vi "ZS_DPLab_Main_ver4.0.vi"() -> ()   [LabVIEW 2012]
panel:
  in  "File type":u16(ring) items=["Txt"=0, "Both"=2]
  out "StartTime(ms)":u32
  in  "Pause":bool
  in  "stop":bool
  in  "Main Sweep":u8(ring) items=["Time", "DC Current", "Delta Current", "Pulse Delta Current", "Sine Current", "Lock-In Vosc"]
  out "Run index":string
  in  "File Index:":u16=1 format="%03d"
  out "TakingData":bool
  in  "Data File Address":path
  in  "Tab Control":T1(tab)
  in  "Steps Config:":T2={"# of points:"=100, "Step Delay (s)"=1.0, "Ini Delay (s)"=3.0, "# of steps:"=1} {"# of steps:" step=1; "# of points:" step=1; "Step Delay (s)" min=0.0 format="%3.2f"; "Ini Delay (s)" min=0.0 format="%3.2f"}
  in  "Tab Control 2":enum32{"ITC 503", "LS 340"}(tab)
  in  "Temperature Control (ITC 503):":T3={"GPIB ADR"=0, "Change Heater?"={"Change Heater?"=FALSE, "Heater"=0}, "Change Temp?"={"Change Temp?"=FALSE, "Set Temp (K)"=0.0}, "Cluster"={"Heat Auto?"=FALSE, "Manual Heat?"=FALSE, "Heater Manual (%)"=0.0}, "Change PID?"={"Change PID?"=FALSE, "Proportional"=0.0, "Integral"=0.0, "Derivative"=0.0}, "Change Para?"=FALSE, "ITC503 Control Sensor"=1} {"ITC503 Control Sensor" items=["T2", "T3"]; "Change PID?"."Derivative" format="%.2f"; "Change PID?"."Integral" format="%.2f"; "Change PID?"."Proportional" format="%.2f"; "Cluster"."Heater Manual (%)" scale=0.0..100.0; "Change Temp?"."Set Temp (K)" format="%.3f"; "Change Heater?"."Heater" items=["Heater 1", "Heater 2", "Heater 3"]; "GPIB ADR" items=["None"=0, "24"=24]}
  in  "Temperature Control (LS 340):":T4={"GPIB ADR"=0, "From (K)"=0.0, "To (K)"=0.0, "Rate (K/min; 0~100)"=1.0, "Delta T (0.08K)"=0.08, "Temp. Header"="Temp_K", "Temp. Display controller"={"Ch B"=TRUE, "Ch C"=TRUE, "Ch D"=FALSE}} {"Delta T (0.08K)" format="%.3f"; "Rate (K/min; 0~100)" format="%.1f"; "To (K)" format="%.2f"; "From (K)" format="%.3f"; "GPIB ADR" items=["None"=0, "30"=30, "12"=12]}
  in  "Measuring Instruments :":T5(array[cluster])
  in  "Keithley 6221 :":T6(array[cluster]) {"Sweep Mode" items=["Linear", "Log", "Exp", "Inverse", "Manual"]; "GPIB ADR" items=["None"=0, "12"=12, "13"=13]; "To I_Sin (A)" format="%#.5p"; "To I_H (A)" format="%#.5p"; "To I_HI (A)" format="%#.5p"; "To I (A)" format="%#.5p"; "Delay (s)" format="%.3p"; "Pulse Width (s)" format="%.3p"; "Delay Time (s)" format="%#.5p"; "DC Offset (A)" format="%#.5p"; "From I_Sin (A)" format="%#.5p"; "Freq (Hz)" format="%#_6p"; "I_L (A)" format="%#.5p"; "From I_H (A)" format="%#.5p"; "I_LO (A)" format="%#.5p"; "From I (A)" format="%#.5p"; "From I_HI (A)" format="%#.5p"}
  in  "Lock-In SR7265 :":T7(array[cluster]) {"Sweep Mode" items=["Linear", "Log", "Exp", "Inverse", "Manual"]; "To" format="%#.5p"; "From" format="%#.5p"; "GPIB ADR" items=["None"=0, "11"=11, "16"=16]}
  in  "Description of this measurement":string
  in  "Varialbe Instruments:":i32(listbox)
  in  "Instruments Config:":string[][](table) caption="Table"
  out "Configuration Profile:":string
  in  "Up Button":bool
  in  "Delete Button":bool
  in  "Down Button":bool
  in  "Add one Run":bool
  in  "Tab Control 3":enum32{"ReadMe", "IPS120", "CS4"}(tab)
  in  "Magnet Control (IPS 120-10)":T8={"Action"=1, "Standby (s)"=0.0, "Heater on (s)"=300.0, "Sweep Setup "=[], "GPIB ADR"=0, "Change Para?"=FALSE} {"GPIB ADR" items=["None"=0, "25"=25]; "Sweep Setup"."Hold(min)" min=0.0; "Sweep Setup"."Set Rate(T/min)" min=0.001 max=0.5 step=0.001; "Sweep Setup"."Set Point (T)" min=-9.0 max=9.0 step=0.001; "Action" items=["Hold", "To Set Point", "To Zero", "Clamp"]}
  in  "Magnet Control (CS4)":T9={"Action"=1, "Standby (s)"=0.0, "Heater on (s)"=300.0, "Sweep Setup "=[], "GPIB ADR"=0, "Change Para?"=FALSE} {"GPIB ADR" items=["None"=0, "10"=10]; "Sweep Setup"."Rate in Range (T/min)" min=0.001 max=0.5 step=0.001 format="%_6g"; "Sweep Setup"."Hold(min)" min=0.0; "Sweep Setup"."Set Point (T)" min=-12.0 max=12.0 step=0.001; "Action" items=["Up", "Down", "Pause", "Zero"]}
  in  "SettingGo":bool
  in  "Discarded pts":i32
  in  "Analysis":bool=TRUE
  in  "Measure with H/T sweep?":bool=TRUE
  in  "LS372 Bridge :":T10(array[cluster]) {"Voltage" items=["2.00 uV"=1, "6.32 uV"=2, "20.0 uV"=3, "63.2 uV"=4, "200 uV"=5, "632 uV"=6, "2.0 mV"=7, "6.32 mV"=8]; "Current" items=["1.00 pA"=1, "3.16 pA"=2, "10.0 pA"=3, "31.6 pA"=4, "100 pA"=5, "316 pA"=6, "1.00 nA"=7, "3.16 nA"=8, "10 nA"=9, "31.6 nA"=10, "100 nA"=11, "316 nA"=12, "1.00 uA"=13, "3.16 uA"=14, "10.0 uA"=15, "31.6 uA"=16, "100 uA"=17, "316 uA"=18, "1.00 mA"=19, "3.16 mA"=20, "10.0 mA"=21, "31.6 mA"=22]; "Range (Ohms)" items=["2.0 m"=1, "6.32 m"=2, "20.0 m"=3, "63.2 m"=4, "200 m"=5, "632 m"=6, "2.00"=7, "6.32"=8, "20.0"=9, "63.2"=10, "200"=11, "632"=12, "2.00 k"=13, "6.32 k"=14, "20.0 k"=15, "63.2 k"=16, "200 k"=17, "632 k"=18, "2.00 M"=19, "6.32 M"=20, "20.0 M"=21, "63.2 M"=22]; "Excitation Mode" items=["Voltage", "Current"]; "GPIB ADR" items=["3"=3, "None"=0, "9"=9]}
  in  "Run Batch Array":T11(array[cluster]) {"Magnet Control (CS4) 2"."GPIB ADR" items=["None"=0, "25"=25]; "Magnet Control (CS4) 2"."Sweep Setup"."Rate in Range (T/min)" min=0.001 max=0.5 step=0.001; "Magnet Control (CS4) 2"."Sweep Setup"."Hold(min)" min=0.0; "Magnet Control (CS4) 2"."Sweep Setup"."Set Point (T)" min=-9.0 max=9.0 step=0.001; "Magnet Control (CS4) 2"."Action" items=["Up", "Down", "Pause", "Zero"]; "LS372 Bridge : 2"."Voltage" items=["2.00 uV"=1, "6.32 uV"=2, "20.0 uV"=3, "63.2 uV"=4, "200 uV"=5, "632 uV"=6, "2.0 mV"=7, "6.32 mV"=8]; "LS372 Bridge : 2"."Current" items=["1.00 pA"=1, "3.16 pA"=2, "10.0 pA"=3, "31.6 pA"=4, "100 pA"=5, "316 pA"=6, "1.00 nA"=7, "3.16 nA"=8, "10 nA"=9, "31.6 nA"=10, "100 nA"=11, "316 nA"=12, "1.00 uA"=13, "3.16 uA"=14, "10.0 uA"=15, "31.6 uA"=16, "100 uA"=17, "316 uA"=18, "1.00 mA"=19, "3.16 mA"=20, "10.0 mA"=21, "31.6 mA"=22]; "LS372 Bridge : 2"."Range" items=["2.0 m"=1, "6.32 m"=2, "20.0 m"=3, "63.2 m"=4, "200 m"=5, "632 m"=6, "2.00"=7, "6.32"=8, "20.0"=9, "63.2"=10, "200"=11, "632"=12, "2.00 k"=13, "6.32 k"=14, "20.0 k"=15, "63.2 k"=16, "200 k"=17, "632 k"=18, "2.00 M"=19, "6.32 M"=20, "20.0 M"=21, "63.2 M"=22]; "LS372 Bridge : 2"."Excitation" items=["Voltage", "Current"]; "LS372 Bridge : 2"."GPIB" items=["None"=0, "9"=9]; "Main Sweep" items=["Time", "DC Current", "Delta Current", "Pulse Delta Current", "Sine Current", "Lock-in Vosc"]; "Temperature Control (ITC 503):"."Sensor" items=["T2", "T3"]; "Magnet Control (IPS 120-10)"."Action" items=["Hold", "To Set point", "To Zero", "Clamp"]; "Keithley 6221 :"."Sweep Mode" items=["Linear", "Log", "Exp", "Inverse", "Manual"]}
  in  "Delete Run":bool
  in  "BatchSettingGo":bool
  out "T2":string
  out "T3":string
  out "B":string
  out "T1":string
  in  "DisplayControl":T12 {"Scale" items=["L", "R"]; "Y - axes"."Y 6" items=["", "Time_sec", "Temp_K", "ChC_K", "BField_T", "Rx", "Ry", "Rx", "Ry"]; "Y - axes"."Y 5" items=["", "Time_sec", "Temp_K", "ChC_K", "BField_T", "Rx", "Ry", "Rx", "Ry"]; "Y - axes"."Y 4" items=["", "Time_sec", "Temp_K", "ChC_K", "BField_T", "Rx", "Ry", "Rx", "Ry"]; "Y - axes"."Y 3" items=["", "Time_sec", "Temp_K", "ChC_K", "BField_T", "Rx", "Ry", "Rx", "Ry"]; "Y - axes"."Y 2" items=["", "Time_sec", "Temp_K", "ChC_K", "BField_T", "Rx", "Ry", "Rx", "Ry"]; "Y - axes"."Y 1" items=["", "Time_sec", "Temp_K", "ChC_K", "BField_T", "Rx", "Ry", "Rx", "Ry"]; "X - axis" items=["Time_sec", "Temp_K", "ChC_K", "BField_T", "Rx", "Ry", "Rx", "Ry"]}
  out "XY Graph":cluster{"DataOut":dbl[], "DataOut":dbl[]}[](graph)
  out "DataDisplay":T13
  out "Set T:":string
  out "Set B:":string
  out "Title Name Array":string[](array[string])
  out "Data Table":dbl[][](array[numeric])
  out "XY Graph 2":cluster{"DataOut":dbl[], "DataOut":dbl[]}[](graph)
  in  "AnalysisDisplayControl":T12 {"Scale" items=["L", "R"]; "Y - axes"."Y 6" items=["", "Time_sec", "Temp_K", "ChC_K", "BField_T", "Rx", "Ry", "Rx", "Ry"]; "Y - axes"."Y 5" items=["", "Time_sec", "Temp_K", "ChC_K", "BField_T", "Rx", "Ry", "Rx", "Ry"]; "Y - axes"."Y 4" items=["", "Time_sec", "Temp_K", "ChC_K", "BField_T", "Rx", "Ry", "Rx", "Ry"]; "Y - axes"."Y 3" items=["", "Time_sec", "Temp_K", "ChC_K", "BField_T", "Rx", "Ry", "Rx", "Ry"]; "Y - axes"."Y 2" items=["", "Time_sec", "Temp_K", "ChC_K", "BField_T", "Rx", "Ry", "Rx", "Ry"]; "Y - axes"."Y 1" items=["", "Time_sec", "Temp_K", "ChC_K", "BField_T", "Rx", "Ry", "Rx", "Ry"]; "X - axis" items=["Time_sec", "Temp_K", "ChC_K", "BField_T", "Rx", "Ry", "Rx", "Ry"]}
  in  "Cernox T Fitting Control":T14={"Cernox V title"="CernoxV_V", "Cernox I title"="CernoxI_V", "Cernox V Lockin Sen (V)"=0.001, "Cernox I Lockin Sensitivity (V)"=0.02, "Cernox I Current Amp Sen (A/V)"=1e-05, "Cernox Fit"=FALSE}
  in  "CernoxI measured with a lock-in?":bool
  in  "Cernox_I":dbl=4.965
  # "If set rate = 0,                           Ramping is off."
  # "If set temp. = 0,    \nThe Temp. is not controlled."
  # "Before you start (IPS120):\n1. Check Helium level of the cryostat before you proceed. Generally you should sweep field back to zero if the level is below 16%.\n3. For IPS120, this module is designed for normal sweep mode, so make sure the \"SWITCH HEATER\" is \"SELECT\" and \"CONFIRM\". If you need the persistent mode, please control IPS manualy.\n4. For CS4, the max sweep rates are 0.55 T/min (0 -  7.5 T), 0.37 T/min (7.5 T - 10.5 T), and 0.18 T/min (10.5 T - 12 T).\n5. Recommended B sweep rate is ~ 0.1 T/min."
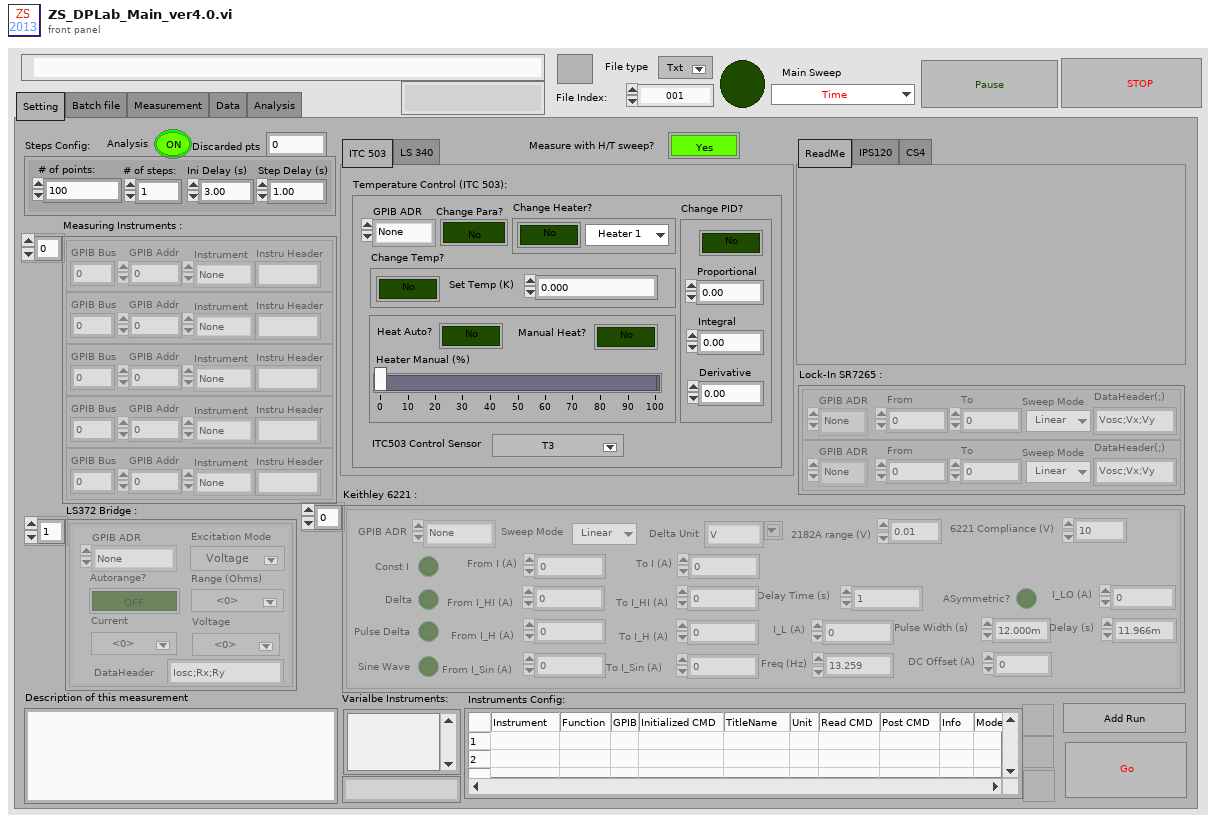
[diagram p1: front panel]
types:
  T1 = enum32{"Setting", "Batch file", "Measurement", "Data", "Analysis"}
  T2 = cluster{"# of points:":u32, "Step Delay (s)":dbl, "Ini Delay (s)":dbl, "# of steps:":u32}
  T3 = cluster{"GPIB ADR":u16, "Change Heater?":cluster{"Change Heater?":bool, "Heater":u8}, "Change Temp?":cluster{"Change Temp?":bool, "Set Temp (K)":dbl}, "Cluster":cluster{"Heat Auto?":bool, "Manual Heat?":bool, "Heater Manual (%)":dbl}, "Change PID?":cluster{"Change PID?":bool, "Proportional":dbl, "Integral":dbl, "Derivative":dbl}, "Change Para?":bool, "ITC503 Control Sensor":u16}
  T4 = cluster{"GPIB ADR":u16, "From (K)":dbl, "To (K)":dbl, "Rate (K/min; 0~100)":dbl, "Delta T (0.08K)":dbl, "Temp. Header":string, "Temp. Display controller":cluster{"Ch B":bool, "Ch C":bool, "Ch D":bool}}
  T5 = cluster{"GPIB Bus":dbl, "GPIB Addr":dbl, "Instrument":enum16{"None", "HP34401DMM", "Lockin 7265", "HP3456/7A", "HP3478A", "HP3325FG", "Keithley2182A"}, "Instru Header":string}[]
  T6 = cluster{"Delta ":bool, "Const I ":bool, "Pulse Delta ":bool, "Sine Wave ":bool, "From I_HI (A)":dbl, "From I (A)":dbl, "I_LO (A)":dbl, "From I_H (A)":dbl, "I_L (A)":dbl, "Freq (Hz)":dbl, "From I_Sin (A)":dbl, "DC Offset (A)":dbl, "Delay Time (s)":dbl, "Pulse Width (s)":dbl, "Delay (s)":dbl, "To I (A)":dbl, "ASymmetric?":bool, "To I_HI (A)":dbl, "To I_H (A)":dbl, "To I_Sin (A)":dbl, "GPIB ADR":u16, "Sweep Mode":u8, "Delta Unit":string, "2182A range (V)":dbl, "6221 Compliance (V)":dbl}[]
  T7 = cluster{"GPIB ADR":u16, "From":dbl, "To":dbl, "DataHeader(;)":string, "Sweep Mode":u8}[]
  T8 = cluster{"Action":u16, "Standby (s)":dbl, "Heater on (s)":dbl, "Sweep Setup ":cluster{"Set Point (T)":dbl, "Set Rate(T/min)":dbl, "Hold(min)":dbl}[], "GPIB ADR":u16, "Change Para?":bool}
  T9 = cluster{"Action":u16, "Standby (s)":dbl, "Heater on (s)":dbl, "Sweep Setup ":cluster{"Set Point (T)":dbl, "Hold(min)":dbl, "Rate in Range (T/min)":dbl[]}[], "GPIB ADR":u16, "Change Para?":bool}
  T10 = cluster{"GPIB ADR":u16, "Excitation Mode":u16, "Autorange?":bool, "Range (Ohms)":u16, "Current":u16, "Voltage":u16, "DataHeader":string}[]
  T11 = cluster{"Main Sweep":u8, "Steps Config:":cluster{"total points:":u32, "Step Delay (s)":dbl, "Ini Delay (s)":dbl, "# of steps:":u32}, "Temperature Control (ITC 503):":cluster{"GPIB ADR":u16, "Change Heater?":cluster{"Heater?":bool, "Heater":u8}, "Change Temp?":cluster{"Change T?":bool, "Set T (K)":dbl}, "Cluster":cluster{"Heat Auto?":bool, "Manual Heat?":bool, "Heater (%)":dbl}, "Change PID?":cluster{"Change PID?":bool, "P":dbl, "I":dbl, "D":dbl}, "Change Para?":bool, "Sensor":u16}, "Temperature Control (LS 340):":cluster{"GPIB ADR":u16, "From (K)":dbl, "To (K)":dbl, "Rate (K/min)":dbl, "Delta T (0.08K)":dbl, "Temp. Header":string, "T Display Control":cluster{"Ch B":bool, "Ch C":bool, "Ch D":bool}}, "Magnet Control (IPS 120-10)":cluster{"Action":u16, "Standby (s)":dbl, "Heater on (s)":dbl, "Sweep Setup ":cluster{"Set Point (T)":dbl, "Set Rate(T/min)":dbl, "Hold(min)":dbl}[], "GPIB ADR":u16, "Change Para?":bool}, "Keithley 6221 :":cluster{"Delta mode":bool, "Const I":bool, "Pulse Delta mode":bool, "Sine Wave Mode":bool, "From I_HI (A)":dbl, "From I (A)":dbl, "I_LO (A)":dbl, "From I_H (A)":dbl, "I_L (A)":dbl, "Freq (Hz)":dbl, "From I_Sin (A)":dbl, "DC Offset (A)":dbl, "Delay Time (s)":dbl, "Pulse Width (s)":dbl, "Delay (s)":dbl, "To I (A)":dbl, "ASymmetric?":bool, "To I_HI (A)":dbl, "To I_H (A)":dbl, "To I_Sin (A)":dbl, "GPIB ADR":u16, "Sweep Mode":u8, "Delta Unit":string, "2182A range (V)":dbl, "6221 Compliance (V)":dbl}[], "Measuring Instruments : ":cluster{"GPIB Bus":dbl, "GPIB Addr":dbl, "Instrument":enum16{"None", "HP34401DMM", "Lockin 7265", "HP3456/7A", "HP3478A", "HP3325FG", "Keithley2182A"}, "Instru Header":string}[], "Lock-In SR7265 :":cluster{"GPIB ADR":u16, "From":dbl, "To":dbl, "Header(;)":string, "Sweep Mode":u8}[], "Deascription of \nthis measurement":string, "Instruments Config:":string[][], "LS372 Bridge : 2":cluster{"GPIB":u16, "Excitation":u16, "Autorange?":bool, "Range":u16, "Current":u16, "Voltage":u16, "DataHeader":string}[], "Magnet Control (CS4) 2":cluster{"Action":u16, "Standby (s)":dbl, "Heater on (s)":dbl, "Sweep Setup ":cluster{"Set Point (T)":dbl, "Hold(min)":dbl, "Rate in Range (T/min)":dbl[]}[], "GPIB ADR":u16, "Change Para?":bool}}[]
  T12 = cluster{"X - axis":u8, "Y - axes":cluster{"Y 1":u8, "Y 2":u8, "Y 3":u8, "Y 4":u8, "Y 5":u8, "Y 6":u8}, "Scale":u16[]}
  T13 = cluster{"X":dbl, "Y 1":dbl, "Y 2":dbl, "Y 3":dbl, "Y 4":dbl, "Y 5":dbl, "Y 6":dbl}
  T14 = cluster{"Cernox V title":string, "Cernox I title":string, "Cernox V Lockin Sen (V)":dbl, "Cernox I Lockin Sensitivity (V)":dbl, "Cernox I Current Amp Sen (A/V)":dbl, "Cernox Fit":bool}
  T15 = cluster{"Main Sweep":u8, "Steps Config:":cluster{"total points:":u32, "Step Delay (s)":dbl, "Ini Delay (s)":dbl, "# of steps:":u32}, "Temperature Control (ITC 503):":cluster{"GPIB ADR":u16, "Change Heater?":cluster{"Heater?":bool, "Heater":u8}, "Change Temp?":cluster{"Change T?":bool, "Set T (K)":dbl}, "Cluster":cluster{"Heat Auto?":bool, "Manual Heat?":bool, "Heater (%)":dbl}, "Change PID?":cluster{"Change PID?":bool, "P":dbl, "I":dbl, "D":dbl}, "Change Para?":bool, "Sensor":u16}, "Temperature Control (LS 340):":cluster{"GPIB ADR":u16, "From (K)":dbl, "To (K)":dbl, "Rate (K/min)":dbl, "Delta T (0.08K)":dbl, "Temp. Header":string, "T Display Control":cluster{"Ch B":bool, "Ch C":bool, "Ch D":bool}}, "Magnet Control (IPS 120-10)":cluster{"Action":u16, "Standby (s)":dbl, "Heater on (s)":dbl, "Sweep Setup ":cluster{"Set Point (T)":dbl, "Set Rate(T/min)":dbl, "Hold(min)":dbl}[], "GPIB ADR":u16, "Change Para?":bool}, "Keithley 6221 :":cluster{"Delta mode":bool, "Const I":bool, "Pulse Delta mode":bool, "Sine Wave Mode":bool, "From I_HI (A)":dbl, "From I (A)":dbl, "I_LO (A)":dbl, "From I_H (A)":dbl, "I_L (A)":dbl, "Freq (Hz)":dbl, "From I_Sin (A)":dbl, "DC Offset (A)":dbl, "Delay Time (s)":dbl, "Pulse Width (s)":dbl, "Delay (s)":dbl, "To I (A)":dbl, "ASymmetric?":bool, "To I_HI (A)":dbl, "To I_H (A)":dbl, "To I_Sin (A)":dbl, "GPIB ADR":u16, "Sweep Mode":u8, "Delta Unit":string, "2182A range (V)":dbl, "6221 Compliance (V)":dbl}[], "Measuring Instruments : ":cluster{"GPIB Bus":dbl, "GPIB Addr":dbl, "Instrument":enum16{"None", "HP34401DMM", "Lockin 7265", "HP3456/7A", "HP3478A", "HP3325FG", "Keithley2182A"}, "Instru Header":string}[], "Lock-In SR7265 :":cluster{"GPIB ADR":u16, "From":dbl, "To":dbl, "Header(;)":string, "Sweep Mode":u8}[], "Deascription of \nthis measurement":string, "Instruments Config:":string[][], "LS372 Bridge : 2":cluster{"GPIB":u16, "Excitation":u16, "Autorange?":bool, "Range":u16, "Current":u16, "Voltage":u16, "DataHeader":string}[], "Magnet Control (CS4) 2":cluster{"Action":u16, "Standby (s)":dbl, "Heater on (s)":dbl, "Sweep Setup ":cluster{"Set Point (T)":dbl, "Hold(min)":dbl, "Rate in Range (T/min)":dbl[]}[], "GPIB ADR":u16, "Change Para?":bool}}
  T16 = enum32{"Setting", "Batch file", "Measurement", "Data"}
  T17 = cluster{"Main Sweep":u8, "Steps Config:":cluster{"# of points:":u32, "Step Delay (s)":dbl, "Ini Delay (s)":dbl, "# of steps:":u32}, "Temperature Control (ITC 503):":cluster{"GPIB ADR":u16, "Change Heater?":cluster{"Change Heater?":bool, "Heater":u8}, "Change Temp?":cluster{"Change Temp?":bool, "Set Temp (K)":dbl}, "Cluster":cluster{"Heat Auto?":bool, "Manual Heat?":bool, "Heater Manual (%)":dbl}, "Change PID?":cluster{"Change PID?":bool, "Proportional":dbl, "Integral":dbl, "Derivative":dbl}, "Change Para?":bool, "ITC503 Control Sensor":u16}, "Temperature Control (LS 340):":cluster{"GPIB ADR":u16, "From (K)":dbl, "To (K)":dbl, "Rate (K/min; 0~100)":dbl, "Delta T (0.08K)":dbl, "Temp. Header":string, "Temp. Display controller":cluster{"Ch B":bool, "Ch C":bool, "Ch D":bool}}, "Magnet Control (IPS 120-10)":cluster{"Action":u16, "Standby (s)":dbl, "Heater on (s)":dbl, "Sweep Setup ":cluster{"Set Point (T)":dbl, "Set Rate(T/min)":dbl, "Hold(min)":dbl}[], "GPIB ADR":u16, "Change Para?":bool}, "Keithley 6221 :":cluster{"Delta ":bool, "Const I ":bool, "Pulse Delta ":bool, "Sine Wave ":bool, "From I_HI (A)":dbl, "From I (A)":dbl, "I_LO (A)":dbl, "From I_H (A)":dbl, "I_L (A)":dbl, "Freq (Hz)":dbl, "From I_Sin (A)":dbl, "DC Offset (A)":dbl, "Delay Time (s)":dbl, "Pulse Width (s)":dbl, "Delay (s)":dbl, "To I (A)":dbl, "ASymmetric?":bool, "To I_HI (A)":dbl, "To I_H (A)":dbl, "To I_Sin (A)":dbl, "GPIB ADR":u16, "Sweep Mode":u8, "Delta Unit":string, "2182A range (V)":dbl, "6221 Compliance (V)":dbl}[], "Measuring Instruments : ":cluster{"GPIB Bus":dbl, "GPIB Addr":dbl, "Instrument":enum16{"None", "HP34401DMM", "Lockin 7265", "HP3456/7A", "HP3478A", "HP3325FG", "Keithley2182A"}, "Instru Header":string}[], "Lock-In SR7265 :":cluster{"GPIB ADR":u16, "From":dbl, "To":dbl, "DataHeader(;)":string, "Sweep Mode":u8}[], "Description of this measurement":string, "Instruments Config:":string[][], "LS372 Bridge :":cluster{"GPIB ADR":u16, "Excitation Mode":u16, "Autorange?":bool, "Range (Ohms)":u16, "Current":u16, "Voltage":u16, "DataHeader":string}[], "Magnet Control (CS4)":cluster{"Action":u16, "Standby (s)":dbl, "Heater on (s)":dbl, "Sweep Setup ":cluster{"Set Point (T)":dbl, "Hold(min)":dbl, "Rate in Range (T/min)":dbl[]}[], "GPIB ADR":u16, "Change Para?":bool}}
  T18 = typedef "LVRowAndColumnTypeDef.ctl" = cluster{"Row":i32, "Column":i32}
  T19 = cluster{"Delta mode":bool, "Const I":bool, "Pulse Delta mode":bool, "Sine Wave Mode":bool, "From I_HI (A)":dbl, "From I (A)":dbl, "I_LO (A)":dbl, "From I_H (A)":dbl, "I_L (A)":dbl, "Freq (Hz)":dbl, "From I_Sin (A)":dbl, "DC Offset (A)":dbl, "Delay Time (s)":dbl, "Pulse Width (s)":dbl, "Delay (s)":dbl, "To I (A)":dbl, "ASymmetric?":bool, "To I_HI (A)":dbl, "To I_H (A)":dbl, "To I_Sin (A)":dbl, "GPIB ADR":u16, "Sweep Mode":u8, "Delta Unit":string, "2182A range (V)":dbl, "6221 Compliance (V)":dbl}[]
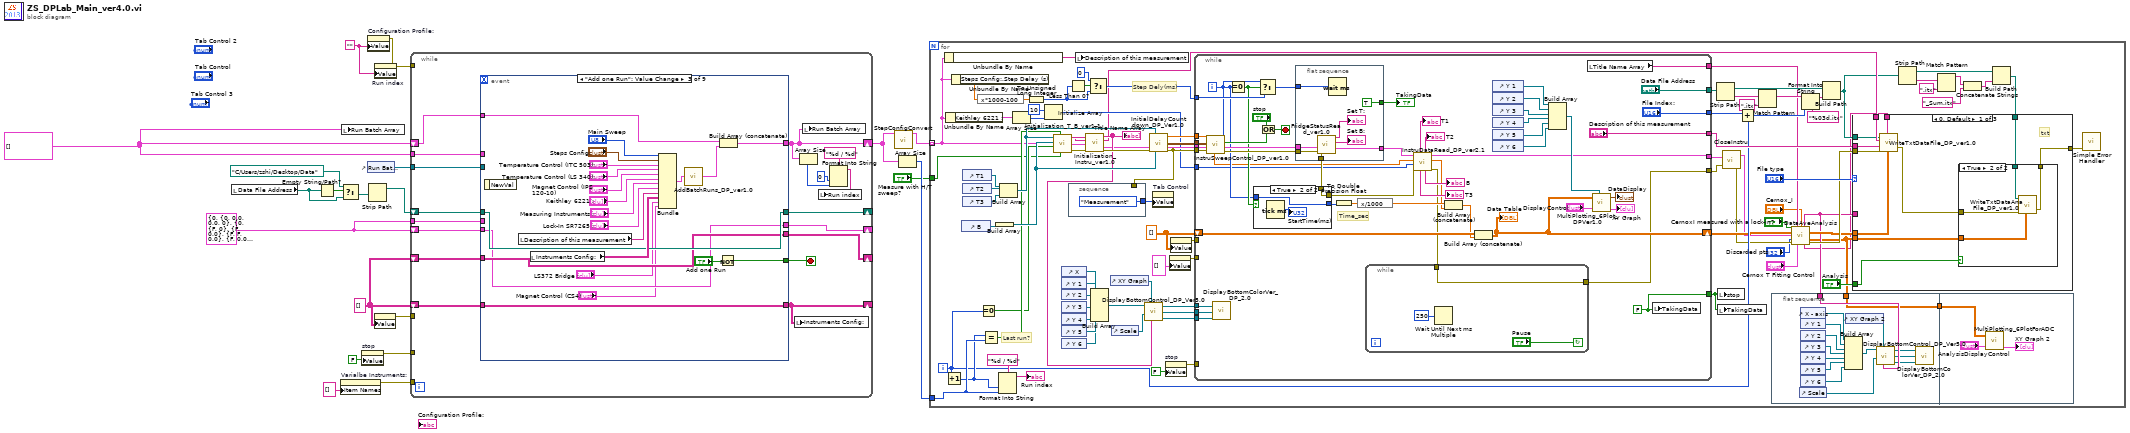
[diagram p0: block diagram]
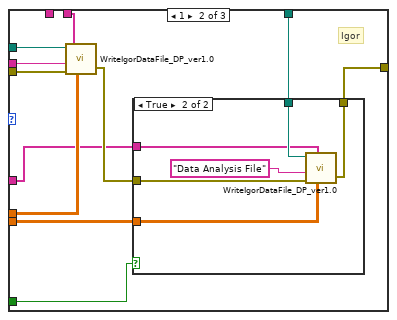
[diagram p3: hidden frame]
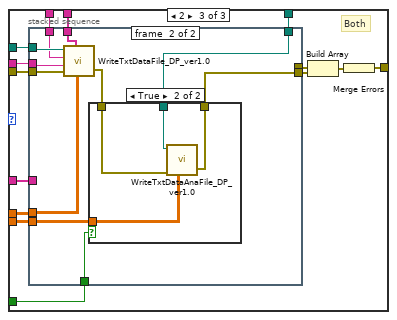
[diagram p5: hidden frame]
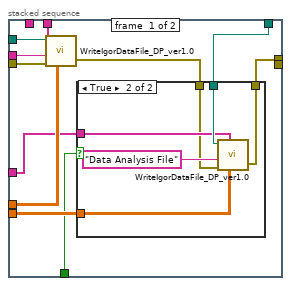
[diagram p6: hidden frame]
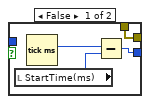
[diagram p9: hidden frame]
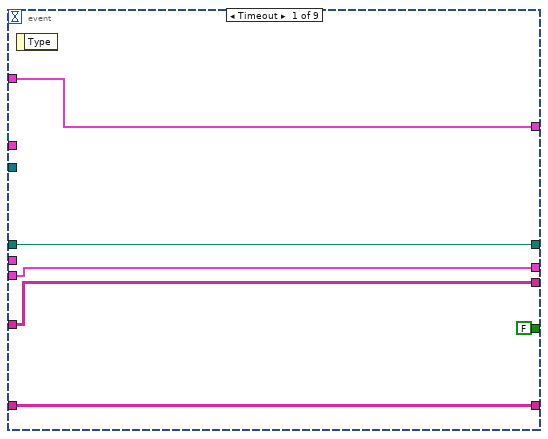
[diagram p10: hidden frame]
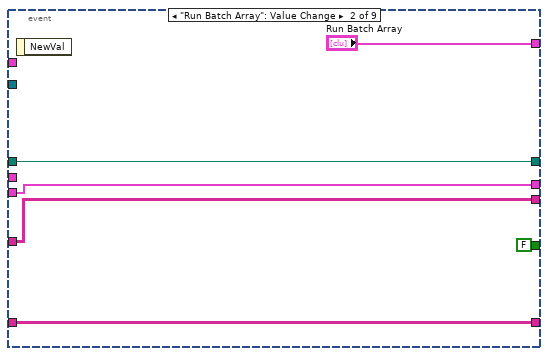
[diagram p11: hidden frame]
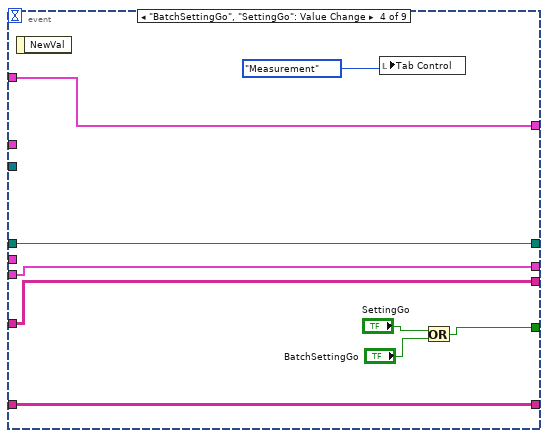
[diagram p12: hidden frame]
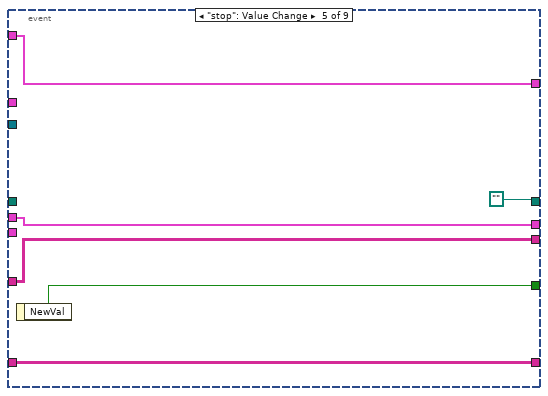
[diagram p13: hidden frame]
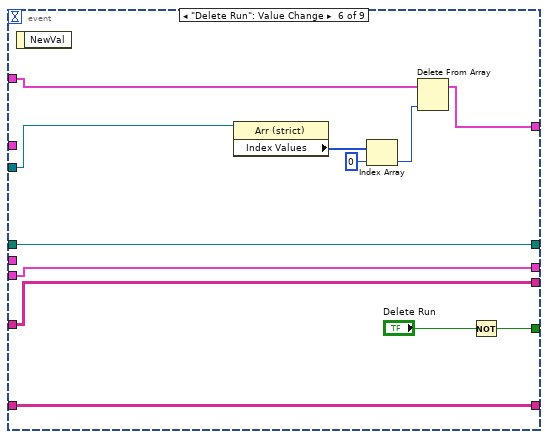
[diagram p14: hidden frame]
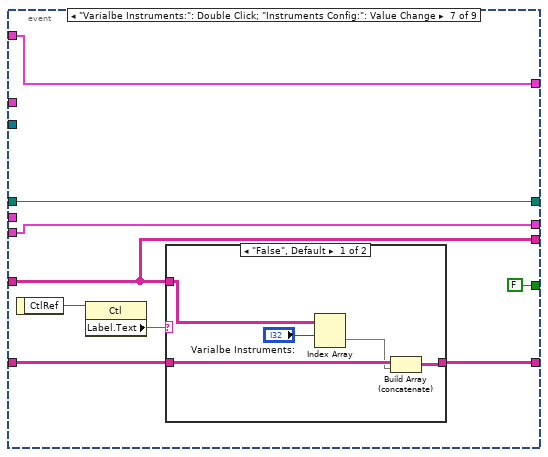
[diagram p15: hidden frame]
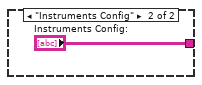
[diagram p16: hidden frame]
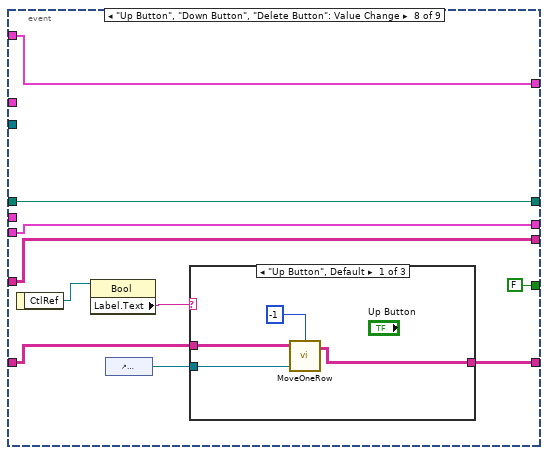
[diagram p17: hidden frame]
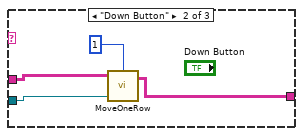
[diagram p18: hidden frame]
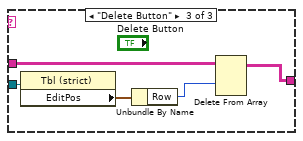
[diagram p19: hidden frame]
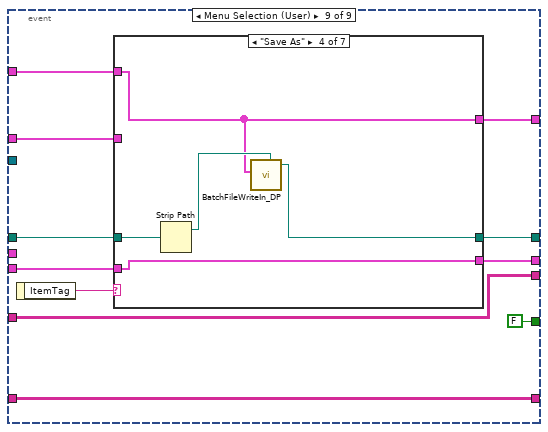
[diagram p20: hidden frame]
diagram:
  w1 = T15 {"Main Sweep"=0, "Steps Config:"={"total points:"=0, "Step Delay (s)"=0.0, "Ini Delay (s)"=0.0, "# of steps:"=0}, "Temperature Control (ITC 503):"={"GPIB ADR"=0, "Change Heater?"={"Heater?"=FALSE, "Heater"=0}, "Change Temp?"={"Change T?"=FALSE, "Set T (K)"=0.0}, "Cluster"={"Heat Auto?"=FALSE, "Manual Heat?"=FALSE, "Heater (%)"=0.0}, "Change PID?"={"Change PID?"=FALSE, "P"=0.0, "I"=0.0, "D"=0.0}, "Change Para?"=FALSE, "Sensor"=1}, "Temperature Control (LS 340):"={"GPIB ADR"=0, "From (K)"=0.0, "To (K)"=0.0, "Rate (K/min)"=0.0, "Delta T (0.08K)"=0.0, "Temp. Header"="", "T Display Control"={"Ch B"=FALSE, "Ch C"=FALSE, "Ch D"=FALSE}}, "Magnet Control (IPS 120-10)"={"Action"=0, "Standby (s)"=0.0, "Heater on (s)"=0.0, "Sweep Setup "=[], "GPIB ADR"=0, "Change Para?"=FALSE}, "Keithley 6221 :"=[], "Measuring Instruments : "=[], "Lock-In SR7265 :"=[], "Deascription of \nthis measurement"="", "Instruments Config:"=[], "LS372 Bridge : 2"=[{"GPIB"=0, "Excitation"=0, "Autorange?"=FALSE, "Range"=0, "Current"=0, "Voltage"=0, "DataHeader"="Rx;Ry"}], "Magnet Control (CS4) 2"={"Action"=1, "Standby (s)"=0.0, "Heater on (s)"=300.0, "Sweep Setup "=[], "GPIB ADR"=0, "Change Para?"=FALSE}} ("output cluster")
  w2 = T11 [] ("Run Batch Array 2")
  w13 = ""
  w19 = string[][] [] ("Instruments Config:")
  n1 = local read "Data File Address"() -> (w16:path)
  n2 = Empty String/Path?(string/path=w16) -> (empty?=w18:bool)
  n3 = property on="Varialbe Instruments:" class="LstBox (strict)"("Item Names"=string[] []) -> (error out=w10:errorcluster)  [unwired: 2 in, 1 out]
  n4 = local write "Run Batch Array"(w2) -> ()
  n5 = Select(t=path "C:/Users/zshi/Desktop/Data" ("Data File Address"), s=w18, f=w16) -> (s? t:f=w15:path)
  n6 = property on="stop" class="Bool (strict)"("Value"=FALSE ("stop")) -> (error out=w6:errorcluster)  [unwired: 2 in, 1 out]
  n7 = control-ref of="Run Batch Array"() -> (w21:refnum<vi>)
  n8 = property on="Configuration Profile:" class="Str"("Value"=w13) -> (error out=w12:errorcluster)  [unwired: 2 in, 1 out]
  n9 = Strip Path(path=w15) -> (stripped path=w14:path)  [unwired: 1 out]
  n10 = property on="Instruments Config:" class="Tbl (strict)"("Value"=w19) -> (error out=w20:errorcluster)  [unwired: 2 in, 1 out]
  n11 = property on="Run index" class="Str"(error in=w12, "Value"=w13) -> (error out=w11:errorcluster)  [unwired: 1 in, 1 out]
  n12 = while {
    shift-right: [w22] -> w5
    shift-left: w2 -> [w38]
    tunnel: w21 -> [w37]
    shift-right: [w36] -> _
    shift-left: w19 -> [w34]
    tunnel: w20 -> [_]
    shift-right: [w33] -> _
    shift-left: w19 -> [w35]
    shift-right: [w27] -> _
    shift-left: w14 -> [w28]
    tunnel: w11 -> [_]
    tunnel: w10 -> [_]
    tunnel: w6 -> [_]
    tunnel: w2 -> [w26]
    shift-right: [w25] -> _
    shift-left: w1 -> [w24]
    tunnel: w1 -> [w23]
    stop <- w39 stop-if-true
    n13 = event shown="[2] \"Add one Run\": Value Change" {
      selector: _ -> [_ _ _ _ _ _ _ _ _]
      dyn-events: _ -> [_ _ _ _ _ _ _ _ _]
      timeout: _ -> [_ _ _ _ _ _ _ _ _]
      tunnel: [FALSE FALSE w63 w79 w88 w99 FALSE ("NewVal") FALSE ("NewVal") FALSE ("NewVal")] -> w39
      tunnel: w38 -> [w44 _ w62 w82 w87 w94 w103 w118 w146]
      tunnel: [w44 "Run Batch Array" w61 w82 w87 w93 w103 w118 w147] -> w22
      tunnel: w37 -> [_ _ _ _ _ w98 _ _ _]
      tunnel: [w41 w47 w58 w76 w85 w90 w107 w119 w140] -> w36
      tunnel: w35 -> [w42 w48 w59 w77 w86 w91 w105 w121 w141]
      tunnel: w34 -> [w41 w47 w58 w76 w85 w90 w106 w120 w140]
      tunnel: [w42 w48 w59 w77 w86 w91 w105 w121 w141] -> w33
      tunnel: w28 -> [w43 w49 w60 w78 _ w92 w102 w117 w145]
      tunnel: [w43 w49 w60 w78 path "" w92 w102 w117 w144] -> w27
      tunnel: w26 -> [_ _ _ _ _ _ _ _ w148]
      tunnel: [w40 w46 w55 w74 w83 w89 w101 w116 w143] -> w25
      tunnel: w24 -> [w40 w46 w55 w74 _ w89 w101 w116 w142]
      tunnel: w23 -> [_ _ _ _ w83 _ _ _ _]
      event Timeout {
        n14 = event-data() -> ()  [unwired: 1 in, 1 out]
      }
      event "Run Batch Array": Value Change {
        n15 = event-data() -> ()  [unwired: 1 in, 1 out]
      }
      event "Add one Run": Value Change {
        n16 = event-data() -> ()  [unwired: 1 in, 1 out]
        n17 = local read "Description of this measurement"() -> (w66:string)
        n18 = local read "Instruments Config:"() -> (w65:string[][])
        n19 = Bundle("Main Sweep"="Main Sweep", "Steps Config:"="Steps Config:", "Temperature Control (ITC 503):"="Temperature Control (ITC 503):", "Temperature Control (LS 340):"="Temperature Control (LS 340):", "Magnet Control (IPS 120-10)"="Magnet Control (IPS 120-10)", "Keithley 6221 :"="Keithley 6221 :", "Measuring Instruments :"="Measuring Instruments :", "Lock-In SR7265 :"="Lock-In SR7265 :", "Description of this measurement"=w66, "Instruments Config:"=w65, "LS372 Bridge :"="LS372 Bridge :", "Magnet Control (CS4)"="Magnet Control (CS4)") -> (w52:T17)  [unwired: 1 in]
        n20 = call "AddBatchRuns_DP_ver1.0.vi"("output cluster"=w52) -> ("output cluster 2"=w57:T15)
        n21 = Not(x="Add one Run") -> (.not. x?=w63:bool)
        n22 = Build Array (concatenate)(w62, w57) -> (w61:T11)
      }
      event "BatchSettingGo", "SettingGo": Value Change {
        n23 = event-data() -> ()  [unwired: 1 in, 1 out]
        n24 = local write "Tab Control"(T16."Measurement" ("Tab Control")) -> ()
        n25 = Or(x="SettingGo", y="BatchSettingGo") -> (x .or. y?=w79:bool)
      }
      event "stop": Value Change {
        n26 = event-data() -> ("NewVal"=w88:bool)  [unwired: 1 in]
      }
      event "Delete Run": Value Change {
        n27 = event-data() -> ()  [unwired: 1 in, 1 out]
        n28 = property class="Arr (strict)"(reference=w98) -> ("Index Values"=w97:u32[])  [unwired: 1 in, 2 out]
        n29 = Index Array(array=w97, index=0) -> (element=w95:u32)
        n30 = Delete From Array(array=w94, index=w95) -> (array with subset deleted=w93:T11)  [unwired: 1 in, 1 out]
        n31 = Not(x="Delete Run") -> (.not. x?=w99:bool)
      }
      event "Varialbe Instruments:": Double Click; "Instruments Config:": Value Change {
        n32 = event-data() -> ("CtlRef"=w109:refnum<vi>)  [unwired: 1 in]
        n33 = property class="Ctl"(reference=w109) -> ("Label.Text"=w108:string)  [unwired: 1 in, 2 out]
        n34 = case shown="\"False\", Default" w108 {
          tunnel: [w110 "Instruments Config:"] -> w107
          tunnel: w105 -> [w114 _]
          tunnel: w106 -> [w112 _]
          frame "False", Default {
            n35 = Index Array(array=w114, index (row)="Varialbe Instruments:") -> (element=w111:string[])  [unwired: 1 in]
            n36 = Build Array (concatenate)(w112, w111) -> (w110:string[][])
          }
          frame "Instruments Config" {
          }
        }
      }
      event "Up Button", "Down Button", "Delete Button": Value Change {
        n37 = event-data() -> ("CtlRef"=w125:refnum<vi>)  [unwired: 1 in]
        n38 = property class="Bool"(reference=w125) -> ("Label.Text"=w124:string)  [unwired: 1 in, 2 out]
        n39 = control-ref of="Instruments Config:"() -> (w123:refnum<vi>)
        n40 = case shown="\"Up Button\", Default" w124 {
          tunnel: w123 -> [w129 w133 w136]
          tunnel: w120 -> [w127 w132 w137]
          tunnel: [w126 w130 w138] -> w119
          frame "Up Button", Default {
            n41 = call "MoveOneRow.vi"("#ofMoveRows"=-1, "Table In Ref"=w129, "Table In"=w127) -> ("Table Out"=w126:string[][])  [unwired: 2 in]
          }
          frame "Down Button" {
            n42 = call "MoveOneRow.vi"("#ofMoveRows"=1, "Table In Ref"=w133, "Table In"=w132) -> ("Table Out"=w130:string[][])  [unwired: 2 in]
          }
          frame "Delete Button" {
            n43 = property class="Tbl (strict)"(reference=w136) -> ("EditPos"=w135:T18)  [unwired: 1 in, 2 out]
            n44 = Unbundle By Name(w135) -> ("Row"=w134:i32)
            n45 = Delete From Array(array=w137, index (row)=w134) -> (array with subset deleted=w138:string[][])  [unwired: 2 in, 1 out]
          }
        }
      }
      event Menu Selection (User) {
        n46 = event-data() -> ("ItemTag"=w149:string)  [unwired: 1 in]
        n47 = case shown="\"Save As\"" w149 {
          tunnel: w148 -> [w153 _ _ _ _ _ _]
          tunnel: [w153 w155 w161 w165 w171 w178 w184] -> w147
          tunnel: w146 -> [_ _ w161 w165 w172 w178 w185]
          tunnel: w145 -> [w152 w159 w163 w168 w169 w176 w182]
          tunnel: [w151 w156 w162 w166 w169 w176 w182] -> w144
          tunnel: [w150 w154 w160 w164 w170 w177 w183] -> w143
          tunnel: w142 -> [w150 w154 w160 w164 _ _ w183]
          frame "New", Default {
            n48 = Strip Path(path=w152) -> (stripped path=w151:path)  [unwired: 1 out]
          }
          frame "Load" {
            n49 = Strip Path(path=w159) -> (stripped path=w157:path)  [unwired: 1 out]
            n50 = call "BatchFileReadOut_DP.vi"("start path"=w157) -> ("Run Batch Array 2"=w155:T11, "File Path"=w156:path)  [unwired: 6 in, 1 out]
            n51 = local write "Tab Control"(T1."Batch file" ("Tab Control")) -> ()
          }
          frame "Save" {
            n52 = call "BatchFileWriteIn_DP.vi"("Run Batch Array 2"=w161, "file path"=w163) -> ("path"=w162:path)  [unwired: 4 in, 2 out]
          }
          frame "Save As" {
            n53 = Strip Path(path=w168) -> (stripped path=w167:path)  [unwired: 1 out]
            n54 = call "BatchFileWriteIn_DP.vi"("start path"=w167, "Run Batch Array 2"=w165) -> ("path"=w166:path)  [unwired: 4 in, 2 out]
          }
          frame "Cut" {
            n55 = property on="Run Batch Array" class="Arr (strict)"() -> ("Index Values"=w173:u32[])  [unwired: 2 in, 2 out]
            n56 = Index Array(array=w173, index=0) -> (element=w174:u32)
            n57 = Delete From Array(array=w172, index=w174) -> (deleted portion=w170:T15, array with subset deleted=w171:T11)  [unwired: 1 in]
          }
          frame "Copy" {
            n58 = property on="Run Batch Array" class="Arr (strict)"() -> ("Index Values"=w180:u32[])  [unwired: 2 in, 2 out]
            n59 = Index Array(array=w180, index=0) -> (element=w179:u32)
            n60 = Index Array(array=w178, index=w179) -> (element=w177:T15)
          }
          frame "Paste" {
            n61 = property on="Run Batch Array" class="Arr (strict)"() -> ("Index Values"=w190:u32[])  [unwired: 2 in, 2 out]
            n62 = Index Array(array=w190, index=0) -> (element=w187:u32)
            n63 = Equal To 0?(x=w187) -> (x = 0?=w189:bool)
            n64 = Increment(x=w187) -> (x+1=w188:u32)
            n65 = Select(t=w187, s=w189, f=w188) -> (s? t:f=w186:u32)
            n66 = Insert Into Array(array=w185, index=w186, new element=w183) -> (w184:T11)
          }
        }
      }
    }
    n67 = local write "Instruments Config:"(w36) -> ()
    n68 = Array Size(array=w22) -> (size(s)=w31:i32)
    n69 = local write "Run Batch Array"(w22) -> ()
    n70 = Format Into String(format string="%d / %d", 0 ("input 1"), w31) -> (resulting string=w29:string)  [unwired: 2 in, 1 out]
    n71 = local write "Run index"(w29) -> ()
  }
  n72 = call "StepConfigConvert.vi"("Run Batch Array 2"=w5) -> ("Run Batch Array 3"=w4:T11)  [unwired: 10 in]
  n73 = Array Size(array=w5) -> (size(s)=w8:i32)
  n74 = for {
    tunnel: w4 -> [w193] mode=indexing
    tunnel: w8 -> [w225]
    tunnel: "Measure with H/T sweep?" -> [w194]
    i -> [w222]
    w268 = dbl[][] []
    # "Last run?"
    # "Step Dely(ms)"
    n75 = Unbundle By Name(w193) -> ("Deascription of \nthis measurement"=w272:string)
    n76 = Increment(x=w222) -> (x+1=w224:i32)
    n77 = Unbundle By Name(w193) -> ("Keithley 6221 :"=w271:T19)
    n78 = Unbundle By Name(w193) -> ("Steps Config:.Step Delay (s)"=w274:dbl)
    n79 = control-ref of="B"() -> (w246:refnum<vi>)
    n80 = control-ref of="T1"() -> (w249:refnum<vi>)
    n81 = control-ref of="T2"() -> (w248:refnum<vi>)
    n82 = control-ref of="T3"() -> (w247:refnum<vi>)
    n83 = expression code="x*1000-100"(w274) -> (w276:dbl)
    n84 = Equal To 0?(x=w222) -> (x = 0?=w221:bool)
    n85 = Equal?(x=w224, y=w225) -> (x = y?=w223:bool)
    n86 = Build Array(w246) -> (w244:refnum<vi>[])
    n87 = Format Into String(format string="%d / %d", w224, w225) -> (resulting string=→"Run index":string)  [unwired: 2 in, 1 out]
    n88 = Build Array(w249, w248, w247) -> (w245:refnum<vi>[])
    n89 = Array Size(array=w271) -> (size(s)=w270:i32)
    n90 = To Unsigned Long Integer(number=w276) -> (unsigned 32bit integer=w277:u32)
    n91 = Initialize Array(10 ("element"), w270) -> (w226:i32[])
    n92 = call "Initialization_T_B_ver1.1.vi"("output cluster"=w193, "Measure with H/T sweep?"=w194, "First run?"=w221, "Last run?"=w223, "B Field Display Tex Array"=w244, "Temp. Display Ref Array"=w245) -> ("error out"=w283:errorcluster, "output cluster 2"=w284:T15, "Title Array"=w285:string[], "Comments String"=w219:string)  [unwired: 1 in]
    n93 = control-ref of="X"() -> (w267:refnum<vi>)
    n94 = control-ref of="Y 1"() -> (w266:refnum<vi>)
    n95 = control-ref of="Y 2"() -> (w265:refnum<vi>)
    n96 = control-ref of="Y 3"() -> (w264:refnum<vi>)
    n97 = control-ref of="Y 4"() -> (w263:refnum<vi>)
    n98 = control-ref of="Y 5"() -> (w262:refnum<vi>)
    n99 = control-ref of="Y 6"() -> (w261:refnum<vi>)
    n100 = Less Than 0?(x=w277) -> (x < 0?=w275:bool)
    n101 = local write "Description of this measurement"(w272) -> ()
    n102 = call "Initialization_Instru_ver1.0.vi"("error in (no error)"=w283, "output cluster"=w284, "Input Comments String"=w219, "T&B Title Array"=w285) -> ("error out"=w282:errorcluster, "output cluster 2"=w192:T15, "Output Comments String"=w218:string, "Title Array"=w227:string[])  [unwired: 1 in]
    "Title Name Array" <- w227
    n103 = Select(t=u32 0 ("unsigned 32bit integer"), s=w275, f=w277) -> (s? t:f=w273:u32)
    n104 = Build Array(w267, w266, w265, w264, w263, w262, w261) -> (w259:refnum<vi>[])
    n105 = control-ref of="XY Graph"() -> (w260:refnum<vi>)
    n106 = control-ref of="Scale"() -> (w258:refnum<vi>)
    n107 = call "DisplayBottomControl_DP_Ver5.0.vi"("Control Ring Array"=w259, "XYGraph Refnum"=w260, "Scale Arr Refnum"=w258, "Title Name Array"=w227) -> ("Y Ref. Output"=w257:refnum<vi>[], "dup Scale Arr Refnum"=w256:refnum<vi>, "XY WFGraph Ref."=w255:refnum<vi>)  [unwired: 2 in]
    n108 = call "InitialDelayCountdown_DP_Ver1.0.vi"("Temp. Display Ref Array"=w245, "output cluster"=w192, "error in"=w282, "B Field Display Tex Array"=w244) -> ("Stay duration pts"=w279:dbl[], "2D Array of DC Source or Lock-In Ctrl Run Cluster"=w281:cluster{"GPIB ADR":u16, "DC St. Pt.":dbl}[][], "output cluster 2"=w280:T15, "error out"=w242:errorcluster)  [unwired: 8 in]
    n109 = stacked-sequence {
      tunnel: [T16."Measurement" ("Tab Control")] -> w243
      tunnel: w242 -> [_]
      frame #0 {
      }
    }
    n110 = property on="Tab Control" class="TabCtl (strict)"("Value"=w243) -> ()  [unwired: 2 in, 2 out]
    n111 = property on="stop" class="Bool (strict)"("Value"=FALSE ("stop")) -> (error out=w252:errorcluster)  [unwired: 2 in, 1 out]
    n112 = property on="XY Graph" class="XYGraph (strict)"("Value"=cluster{"DataOut":dbl[], "DataOut":dbl[]}[] [] ("Value (Signaling)")) -> (error out=w251:errorcluster)  [unwired: 2 in, 1 out]
    n113 = property on="Data Table" class="Arr (strict)"("Value"=w268) -> (error out=w254:errorcluster)  [unwired: 2 in, 1 out]
    n114 = while {
      tunnel: w281 -> [w438]
      tunnel: w280 -> [w437]
      tunnel: w242 -> [w436]
      tunnel: w279 -> [w439]
      tunnel: w273 -> [w433]
      shift-right: [w412] -> w217
      shift-left: w268 -> [w414]
      tunnel: ["Description of this measurement"] -> w231
      tunnel: [w408] -> w211
      tunnel: w257 -> [w407]
      tunnel: w256 -> [w406]
      tunnel: w255 -> [w405]
      tunnel: w254 -> [_]
      tunnel: w252 -> [_]
      tunnel: w251 -> [_]
      tunnel: [w392] -> w229
      tunnel: [w396] -> w241
      tunnel: ["Data File Address"] -> w233
      tunnel: ["File Index:"] -> w232
      tunnel: [w391] -> w228
      tunnel: w226 -> [w389]
      i -> [w426]
      stop <- w434 stop-if-true
      w396 = FALSE
      # "Time_sec"
      n115 = call "InstruSweepControl_DP_ver1.0.vi"("Run Index"=w426, "error in"=w436, "output cluster"=w437, "2D Array of DC Source or Lock-In Ctrl Run Cluster"=w438, "Stay duration pts"=w439) -> ("error out"=w429:errorcluster, "output cluster 2"=w430:T15, "Run Stop?"=w431:bool, "Const I output"=w390:dbl[])  [unwired: 1 in]
      n116 = call "DisplayBottomColorVer_DP_2.0.vi"("WFGraph Ref."=w405, "Scale Arr Refnum"=w406, "Y Ref. Output"=w407) -> ()  [unwired: 3 in]
      n117 = Equal To 0?(x=w426) -> (x = 0?=w427:bool)
      n118 = case shown="True" w427 {
        tunnel: w426 -> [_ w449]
        tunnel: [w444 w449] -> w425
        tunnel: w423 -> [w443 w447]
        tunnel: [w443 w447] -> w422
        frame False {
          n119 = local read "StartTime(ms)"() -> (w445:u32)
          n120 = Tick Count (ms)() -> (millisecond timer value=w446:u32)
          n121 = Subtract(x=w446, y=w445) -> (x-y=w444:u32)
        }
        frame True {
          n122 = Tick Count (ms)() -> (millisecond timer value=→"StartTime(ms)":u32)
        }
      }
      n123 = Select(t=w426, s=w427, f=w433) -> (s? t:f=w432:u32)
      n124 = Or(x="stop", y=w431) -> (x .or. y?=w434:bool)
      n125 = flat-sequence {
        tunnel: w432 -> [w457]
        tunnel: w430 -> [w455]
        tunnel: w429 -> [w454]
        tunnel: [TRUE] -> w428
        tunnel: [w453] -> w421
        tunnel: [w452] -> w423
        frame #0 {
          n126 = call "FridgeStatusRead_ver1.0.vi"("error in"=w454, "output cluster"=w455) -> ("error out"=w452:errorcluster, "output cluster 2"=w453:T15, "Set B (T)"=→"Set B:":string, "Set T (K)"=→"Set T:":string)  [unwired: 2 in, 4 out]
          n127 = Wait (ms)(milliseconds to wait=w457) -> ()  [unwired: 1 out]
        }
      }
      n128 = To Double Precision Float(number=w425) -> (double precision float=w424:dbl)
      n129 = expression code="x/1000"(w424) -> (w416:dbl)
      n130 = call "InstruDataRead_DP_ver2.1.vi"("error in"=w422, "memory of # of pts in buffer"=w389, "Const I output"=w390, "output cluster"=w421) -> ("error out"=w393:errorcluster, "Data"=w415:dbl[], "output cluster 2"=w391:T15, "B (T)"=→"B":string, "T2 (K)"=→"T2":string, "T3 (K)"=→"T3":string, "T1 (K)"=→"T1":string)  [unwired: 1 out]
      n131 = while {
        tunnel: w393 -> [w442]
        tunnel: [w442] -> w392
        stop <- "Pause" continue-if-true
        n132 = Wait Until Next ms Multiple(millisecond multiple=u32 250) -> ()  [unwired: 1 out]
      }
      n133 = Build Array (concatenate)(w416, w415) -> (w413:dbl[])
      n134 = Build Array (concatenate)(w414, w413) -> (w412:dbl[][])
      "Data Table" <- w412
      n135 = control-ref of="Y 1"() -> (w399:refnum<vi>)
      n136 = control-ref of="Y 2"() -> (w400:refnum<vi>)
      n137 = control-ref of="Y 3"() -> (w401:refnum<vi>)
      n138 = control-ref of="Y 4"() -> (w402:refnum<vi>)
      n139 = control-ref of="Y 5"() -> (w403:refnum<vi>)
      n140 = control-ref of="Y 6"() -> (w404:refnum<vi>)
      n141 = Build Array(w399, w400, w401, w402, w403, w404) -> (w398:refnum<vi>[])
      n142 = local read "Title Name Array"() -> (w408:string[])
      n143 = call "MultiPlotting_6Plot_DPVer1.0.vi"("2D-DataIn"=w412, "DataDisplay Ref Array"=w398, "DisplayControl"="DisplayControl") -> ("DataDisplay"=→"DataDisplay":T13, "XY Graph"=→"XY Graph":cluster{"DataOut":dbl[], "DataOut":dbl[]}[])  [unwired: 3 in]
      n144 = local write "TakingData"(w396) -> ()
      "TakingData" <- w428
    }
    n145 = Strip Path(path=w233) -> (stripped path=w238:path, name=w237:string)
    n146 = local write "stop"(w241) -> ()
    n147 = local write "TakingData"(w241) -> ()
    n148 = call "CloseInstru.vi"("error in"=w229, "output cluster"=w228) -> ("error out"=w214:errorcluster, "output cluster 2"=w216:T15)
    n149 = Add(x=w232, y=w222) -> (x+y=w234:i32)
    n150 = Match Pattern(string=w237, regular expression=".itx") -> (before substring=w235:string)  [unwired: 1 in, 3 out]
    n151 = flat-sequence {
      tunnel: w201 -> [w292]
      tunnel: w200 -> [w288]
      tunnel: [w288] -> w199
      tunnel: w199 -> [w303]
      frame #0 {
        n152 = control-ref of="Scale"() -> (w293:refnum<vi>)
        n153 = control-ref of="X - axis"() -> (w302:refnum<vi>)
        n154 = control-ref of="Y 1"() -> (w301:refnum<vi>)
        n155 = control-ref of="Y 2"() -> (w300:refnum<vi>)
        n156 = control-ref of="Y 3"() -> (w299:refnum<vi>)
        n157 = control-ref of="Y 4"() -> (w298:refnum<vi>)
        n158 = control-ref of="Y 5"() -> (w297:refnum<vi>)
        n159 = control-ref of="Y 6"() -> (w296:refnum<vi>)
        n160 = Build Array(w302, w301, w300, w299, w298, w297, w296) -> (w294:refnum<vi>[])
        n161 = control-ref of="XY Graph 2"() -> (w295:refnum<vi>)
        n162 = call "DisplayBottomControl_DP_Ver5.0.vi"("Control Ring Array"=w294, "XYGraph Refnum"=w295, "Scale Arr Refnum"=w293, "Title Name Array"=w292) -> ("Y Ref. Output"=w291:refnum<vi>[], "dup Scale Arr Refnum"=w290:refnum<vi>, "XY WFGraph Ref."=w289:refnum<vi>)  [unwired: 2 in]
        n163 = call "DisplayBottomColorVer_DP_2.0.vi"("WFGraph Ref."=w289, "Scale Arr Refnum"=w290, "Y Ref. Output"=w291) -> ()  [unwired: 3 in]
      }
      frame #1 {
        n164 = call "MultiPlotting_6PlotForADC.vi"("2D-DataIn"=w303, "DisplayControl"="AnalysisDisplayControl") -> ("XY Graph"=→"XY Graph 2":cluster{"DataOut":dbl[], "DataOut":dbl[]}[])  [unwired: 4 in, 1 out]
      }
    }
    n165 = call "DataAveAnalysis.vi"("CernoxI measured with a lock-in?"="CernoxI measured with a lock-in?", "Title Name Array In"=w211, "Cernox_I"="Cernox_I", "2D Data Array In"=w217, "output cluster"=w216, "# of Discarded pts"="Discarded pts", "error in"=w214, "Cernox T Fitting Control"="Cernox T Fitting Control") -> ("Title Name Array Out"=w201:string[], "2D Data ArrayOut"=w212:dbl[][], "2D Data  Analysis"=w200:dbl[][], "Title Name Before Std"=w197:string[], "error out"=w215:errorcluster)  [unwired: 2 in, 1 out]
    n166 = Format Into String(format string="%03d.itx", initial string=w235, w234) -> (resulting string=w239:string)  [unwired: 1 in, 1 out]
    n167 = Build Path(base path=w238, name or relative path=w239) -> (appended path=w204:path)
    n168 = Strip Path(path=w204) -> (stripped path=w207:path, name=w205:string)
    n169 = Match Pattern(string=w205, regular expression=".itx") -> (before substring=w208:string)  [unwired: 1 in, 3 out]
    n170 = Concatenate Strings(w208, "_Sum.itx" ("regular expression")) -> (w210:string)
    n171 = Build Path(base path=w207, name or relative path=w210) -> (appended path=w203:path)
    n172 = case shown="0, Default" "File type" {
      tunnel: w204 -> [w312 w332 w353]
      tunnel: w197 -> [w311 w331 w352]
      tunnel: w231 -> [w316 w330 w351]
      tunnel: [w309 w325 w346] -> w230
      tunnel: w215 -> [w315 w329 w350]
      tunnel: w218 -> [w314 _ w349]
      tunnel: w212 -> [w313 w328 w345]
      tunnel: w201 -> [_ w323 w343]
      tunnel: w200 -> [w308 w324 w342]
      tunnel: w203 -> [w307 w327 w344]
      tunnel: "Analysis" -> [w306 w322 w340]
      frame 0, Default {
        # "txt"
        n173 = call "WriteTxtDataFile_DP_ver1.0.vi"("2D Data Array In"=w313, "Title Name Array"=w311, "error in"=w315, "Run Info. Comment"=w316, "Initial String"=w314, "file path"=w312) -> ("error out"=w310:errorcluster)  [unwired: 1 in]
        n174 = case shown="True" w306 {
          tunnel: w310 -> [w317 w321]
          tunnel: [w317 w320] -> w309
          tunnel: w308 -> [_ w319]
          tunnel: w307 -> [_ w318]
          frame False {
          }
          frame True {
            n175 = call "WriteTxtDataAnaFile_DP_ver1.0.vi"("2D Data Array In"=w319, "error in"=w321, "file path"=w318) -> ("error out"=w320:errorcluster)  [unwired: 4 in]
          }
        }
      }
      frame 1 {
        # "Igor"
        n176 = call "WriteIgorDataFile_DP_ver1.0.vi"("2D Data Array In"=w328, "Title Name Array"=w331, "error in"=w329, "Run Info. Comment"=w330, "file path"=w332) -> ("error out"=w326:errorcluster)  [unwired: 2 in]
        n177 = case shown="True" w322 {
          tunnel: w327 -> [_ w339]
          tunnel: w326 -> [w333 w338]
          tunnel: [w333 w337] -> w325
          tunnel: w324 -> [_ w336]
          tunnel: w323 -> [_ w335]
          frame False {
          }
          frame True {
            n178 = call "WriteIgorDataFile_DP_ver1.0.vi"("2D Data Array In"=w336, "Title Name Array"=w335, "error in"=w338, "Run Info. Comment"="Data Analysis File", "file path"=w339) -> ("error out"=w337:errorcluster)  [unwired: 2 in]
          }
        }
      }
      frame 2 {
        # "Both"
        n179 = stacked-sequence {
          tunnel: w353 -> [w364 w381]
          tunnel: w352 -> [w363 w382]
          tunnel: w351 -> [w362 w379]
          tunnel: [w356 _] -> w347
          tunnel: w350 -> [w361 w378]
          tunnel: w349 -> [_ w380]
          tunnel: w345 -> [w360 w377]
          tunnel: w344 -> [w358 w376]
          tunnel: w343 -> [w357 _]
          tunnel: w342 -> [w359 w373]
          tunnel: [_ w374] -> w341
          tunnel: w340 -> [w354 w372]
          frame #0 {
            n180 = call "WriteIgorDataFile_DP_ver1.0.vi"("2D Data Array In"=w360, "Title Name Array"=w363, "error in"=w361, "Run Info. Comment"=w362, "file path"=w364) -> ("error out"=w355:errorcluster)  [unwired: 2 in]
            n181 = case shown="True" w354 {
              tunnel: w359 -> [_ w370]
              tunnel: w358 -> [_ w369]
              tunnel: w357 -> [_ w368]
              tunnel: [w365 w367] -> w356
              tunnel: w355 -> [w365 w366]
              frame False {
              }
              frame True {
                n182 = call "WriteIgorDataFile_DP_ver1.0.vi"("2D Data Array In"=w370, "Title Name Array"=w368, "error in"=w366, "Run Info. Comment"="Data Analysis File", "file path"=w369) -> ("error out"=w367:errorcluster)  [unwired: 2 in]
              }
            }
          }
          frame #1 {
            n183 = call "WriteTxtDataFile_DP_ver1.0.vi"("2D Data Array In"=w377, "Title Name Array"=w382, "error in"=w378, "Run Info. Comment"=w379, "Initial String"=w380, "file path"=w381) -> ("error out"=w375:errorcluster)  [unwired: 1 in]
            n184 = case shown="True" w372 {
              tunnel: w376 -> [_ w387]
              tunnel: w375 -> [w383 w386]
              tunnel: [w383 w385] -> w374
              tunnel: w373 -> [_ w384]
              frame False {
              }
              frame True {
                n185 = call "WriteTxtDataAnaFile_DP_ver1.0.vi"("2D Data Array In"=w384, "error in"=w386, "file path"=w387) -> ("error out"=w385:errorcluster)  [unwired: 4 in]
              }
            }
          }
        }
        n186 = Build Array(w347, w341) -> (w348:errorcluster[])
        n187 = Merge Errors(w348) -> (w346:errorcluster)
      }
    }
    n188 = call <vilib>:"Simple Error Handler.vi"("error in (no error)"=w230) -> ()  [unwired: 4 in, 5 out]
  }
